vi "loadFile.vi"() -> ()   [LabVIEW 2018]
uses:
  <vilib>/Utility/file.llb/Read Delimited Spreadsheet (string).vi
panel:
  in  "openFile":path caption="Open File"
  out "dataGraph":cluster{"X":dbl[], "Y":dbl[]}(graph)
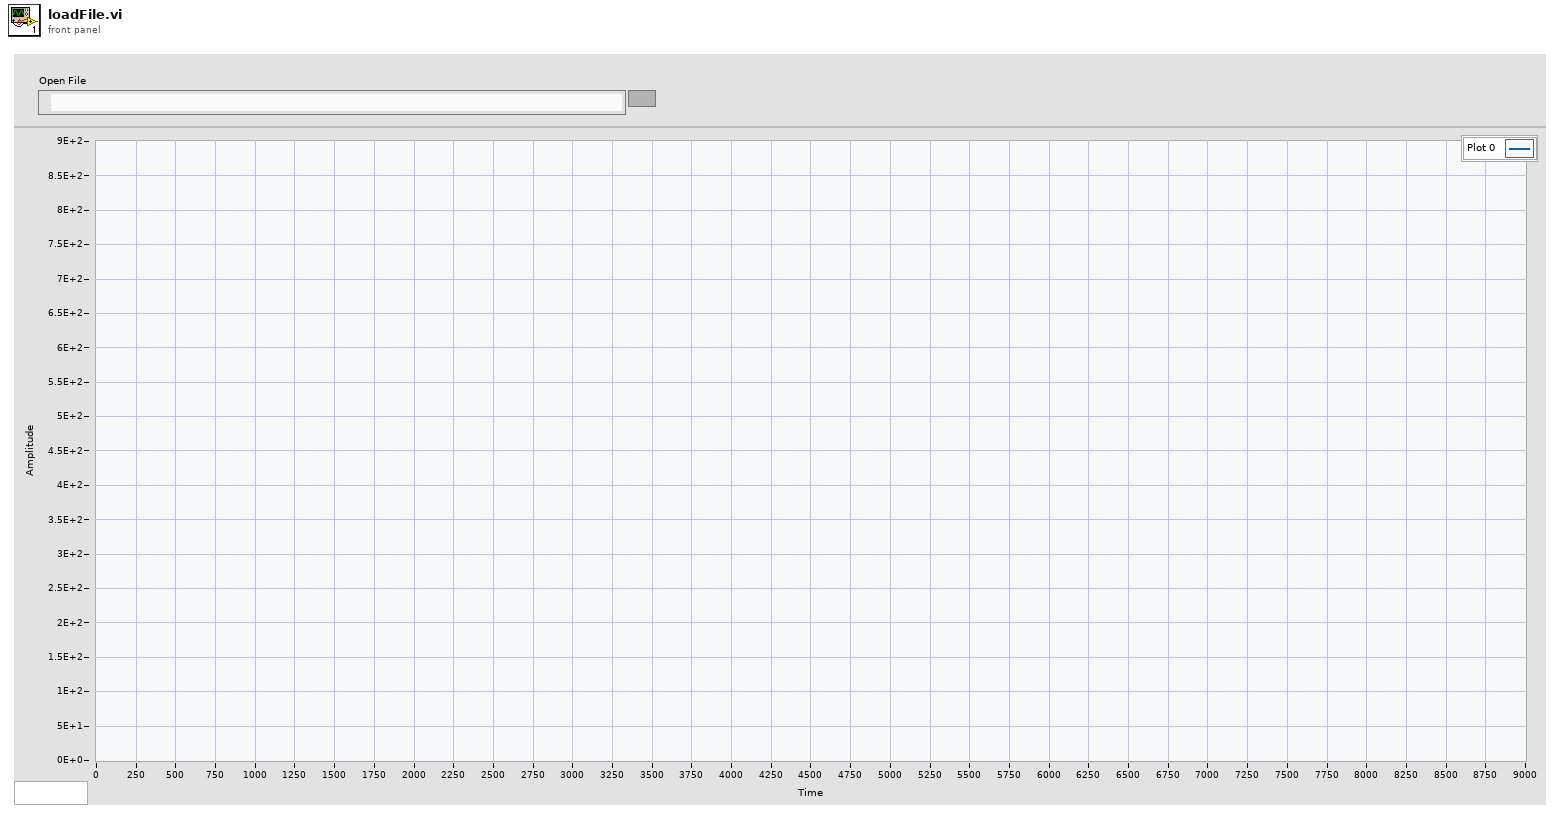
[diagram p1: front panel]
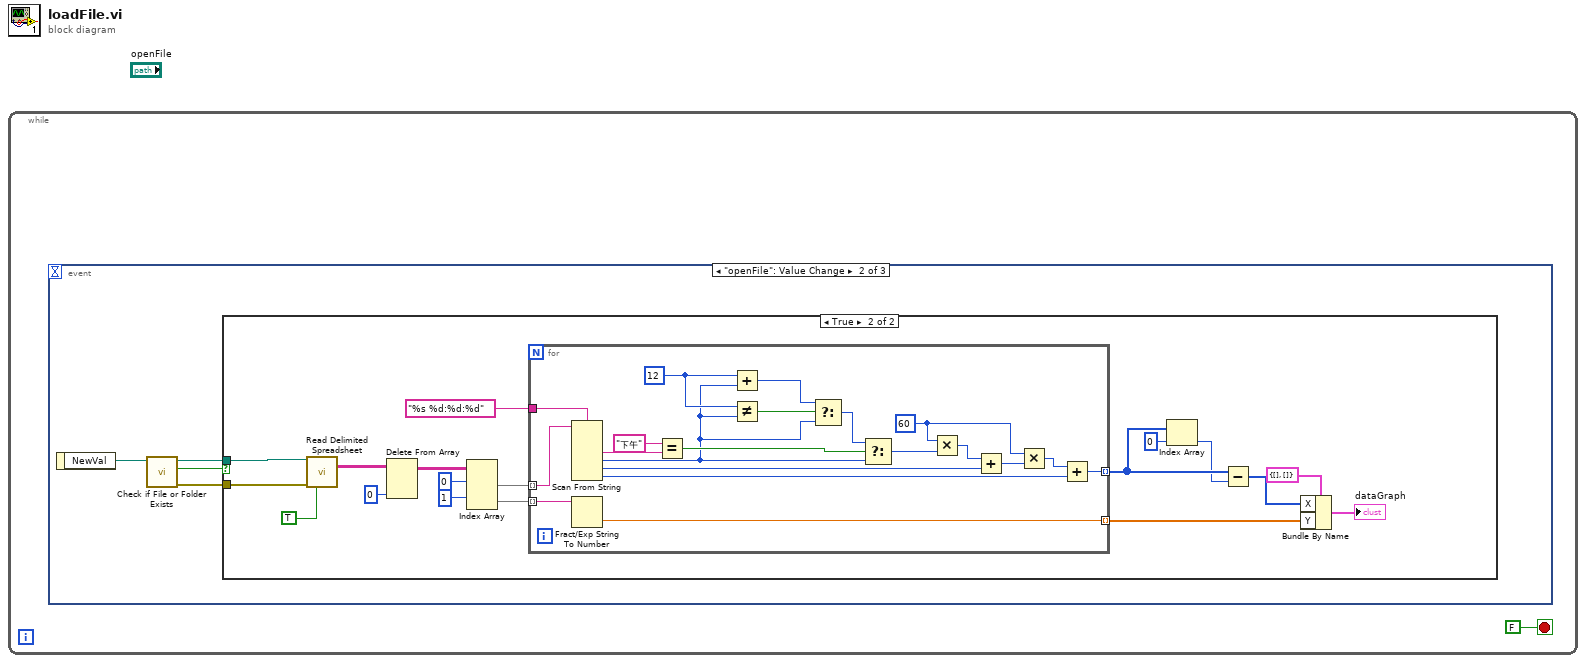
[diagram p0: block diagram]
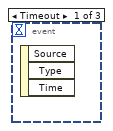
[diagram p2: hidden frame]
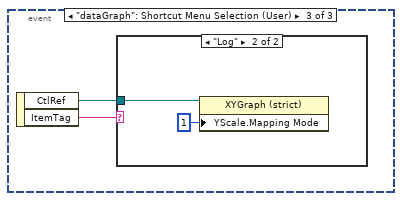
[diagram p4: hidden frame]
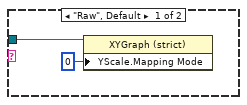
[diagram p5: hidden frame]
diagram:
  n1 = while {
    stop <- FALSE stop-if-true
    n2 = event shown="[1] \"openFile\": Value Change" {
      selector: _ -> [_ _ _]
      dyn-events: _ -> [_ _ _]
      timeout: _ -> [_ _ _]
      event Timeout {
        n3 = event-data() -> ()  [unwired: 1 in, 3 out]
      }
      event "openFile": Value Change {
        n4 = event-data() -> ("NewVal"=w5:path)  [unwired: 1 in]
        n5 = call <vilib>:"Check if File or Folder Exists.vi"("path"=w5) -> ("error out"=w2:errorcluster, "file or folder exists?"=w4:bool, "dup path"=w3:path)  [unwired: 8 in]
        n6 = case shown="True" w4 {
          tunnel: w3 -> [_ w23]
          tunnel: w2 -> [_ w22]
          frame False {
          }
          frame True {
            n7 = call-poly <vilib>:"Read Delimited Spreadsheet.vi"("file path (dialog if empty)"=w23, "error in (no error)"=w22, "transpose? (F)"=TRUE) -> ("all rows"=w20:string[][])  [unwired: 7 in, 5 out]
            n8 = Delete From Array(array=w20, index (col)=0 ("disabled index (col)")) -> (array with subset deleted=w16:string[][])  [unwired: 2 in, 1 out]
            n9 = Index Array(array=w16, index (row) #1=0 ("disabled index (col)"), index (row) #2=1 ("index (col)")) -> (element #1=w15:string[], element #2=w14:string[])  [unwired: 2 in]
            n10 = for {
              tunnel: w15 -> [w30] mode=indexing
              tunnel: w14 -> [w43] mode=indexing
              tunnel: [w29] -> w12 mode=indexing
              tunnel: [w42] -> w6 mode=indexing
              tunnel: "%s %d:%d:%d" ("format string") -> [w31]
              w34 = 60 ("x")
              w28 = 12 ("x")
              n11 = Scan From String(format string=w31, input string=w30) -> (output 1=w41:string, output 2=w25:i32, output 3=w37:i32, output 4=w33:i32)  [unwired: 6 in, 3 out]
              n12 = Fract/Exp String To Number(string=w43) -> (number=w42:dbl)  [unwired: 3 in, 1 out]
              n13 = Equal?(x="下午", y=w41) -> (x = y?=w39:bool)
              n14 = Add(x=w28, y=w25) -> (x+y=w26:i32)
              n15 = Not Equal?(x=w28, y=w25) -> (x != y?=w27:bool)
              n16 = Select(t=w26, s=w27, f=w25) -> (s? t:f=w24:i32)
              n17 = Select(t=w24, s=w39, f=w25) -> (s? t:f=w38:i32)
              n18 = Multiply(x=w34, y=w38) -> (x*y=w36:i32)
              n19 = Add(x=w36, y=w37) -> (x+y=w35:i32)
              n20 = Multiply(x=w34, y=w35) -> (x*y=w32:i32)
              n21 = Add(x=w32, y=w33) -> (x+y=w29:i32)
            }
            n22 = Index Array(array=w12, index=0) -> (element=w11:i32)
            n23 = Subtract(x=w12, y=w11) -> (x-y=w9:i32[])
            n24 = Bundle By Name(cluster=cluster{"X":dbl[], "Y":dbl[]} {"X"=[], "Y"=[]}, "X"=w9, "Y"=w6) -> (→"dataGraph":cluster{"X":dbl[], "Y":dbl[]})
          }
        }
      }
      event "dataGraph": Shortcut Menu Selection (User) {
        n25 = event-data() -> ("CtlRef"=w44:refnum<vi>, "ItemTag"=w45:string)  [unwired: 1 in]
        n26 = case shown="\"Log\"" w45 {
          tunnel: w44 -> [w46 w49]
          frame "Raw", Default {
            n27 = property class="XYGraph (strict)"(reference=w46, "YScale.Mapping Mode"=u8 0 ("Y Scale.Mapping Mode")) -> ()  [unwired: 1 in, 2 out]
          }
          frame "Log" {
            n28 = property class="XYGraph (strict)"(reference=w49, "YScale.Mapping Mode"=u8 1 ("Y Scale.Mapping Mode")) -> ()  [unwired: 1 in, 2 out]
          }
        }
      }
    }
  }
